vi "ReadTest (FPGA).vi"() -> ()   [LabVIEW 2012]
panel:
  out "Read uSec":u32
  out "Points Read":i32
  out "Point":cluster{"X":i32, "Y":i32, "Z":i32}
  in  "Stop":bool
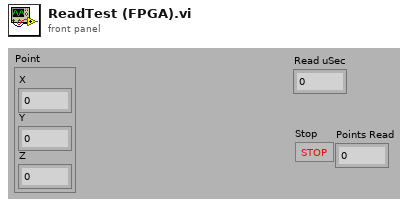
[diagram p1: front panel]
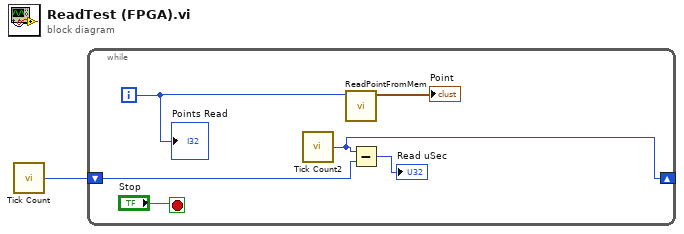
[diagram p0: block diagram]
diagram:
  n1 = call "Tick Count"() -> ("Tick Count(uSec)"=w1:u32)
  n2 = while {
    shift-right: [w3] -> _
    shift-left: w1 -> [w4]
    i -> [w5]
    stop <- "Stop" stop-if-true
    n3 = call "Tick Count2"() -> ("Tick Count(uSec)"=w3:u32)
    n4 = call "ReadPointFromMem.vi"("PointNum"=w5) -> ("Point"=→"Point":cluster{"X":i32, "Y":i32, "Z":i32})  [unwired: 10 in]
    n5 = Subtract(x=w3, y=w4) -> (x-y=→"Read uSec":u32)
    "Points Read" <- w5
  }
